vi "TempForLoop.vi"() -> ()   [LabVIEW 2015]
uses:
  <vilib>/measure/NI_MABase.lvlib
panel:
  out "Hot Temp Change":dbl
  out "Intermediate Temp Change":dbl
  out "Cold Temp Change":dbl
  out "Temperature Changes":cluster{dbl, dbl, dbl}(graph)
  out "Temperature Plot":T1(graph)
  out "Temp Data":T2
  in  "Initial Condition":T3
  in  "?":dbl
  in  "?":dbl
  # "Input desired duration of measurements in seconds"
  # "Input desired Time Measurement Intervals in seconds"
  # "Temperature Change Every Second"
  # "sec"
  # "Deg F"
  # "Deg F"
  # "Deg F"
  # "sed"
  # "Deg F"
  # "Deg F"
  # "Deg F"
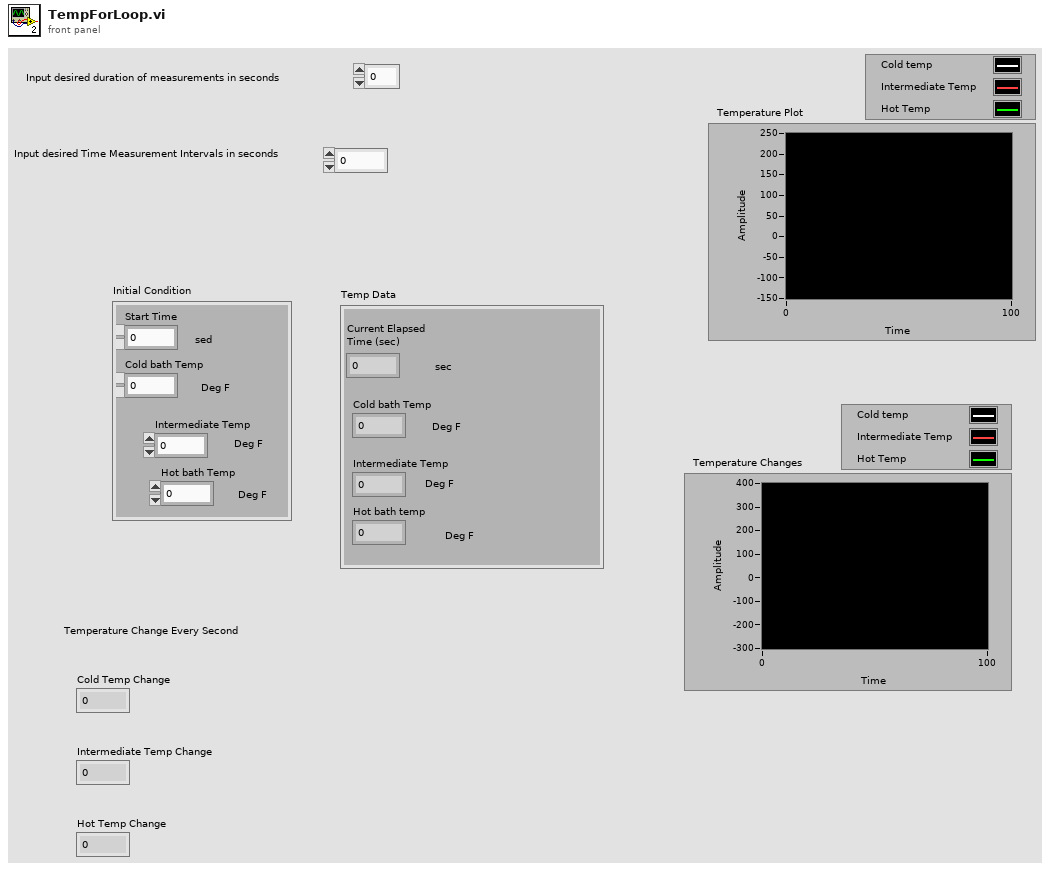
[diagram p1: front panel]
types:
  T1 = cluster{"Cold bath Temp":dbl, "Intermediate Temp":dbl, "Hot bath Temp":dbl}
  T2 = cluster{"Current Elapsed \nTime (sec)":dbl, "Cold bath Temp":dbl, "Intermediate Temp":dbl, "Hot bath temp":dbl}
  T3 = cluster{"Start Time":dbl, "Cold bath Temp":dbl, "Intermediate Temp":dbl, "Hot bath Temp":dbl}
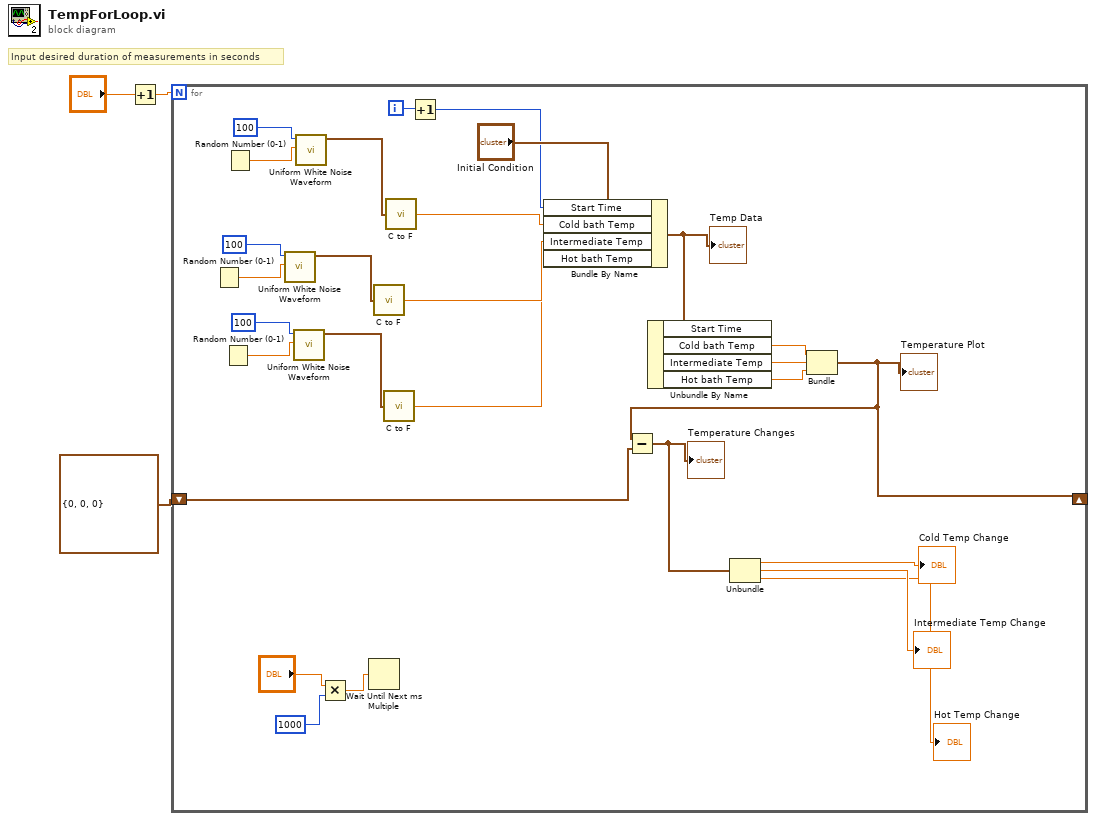
[diagram p0: block diagram]
diagram:
  # "Input desired duration of measurements in seconds"
  n1 = Increment(x="?") -> (x+1=w2:dbl)
  n2 = for {
    N: w2 -> [_]
    shift-right: [w8] -> _
    shift-left: cluster{i32, i32, i32} {0, 0, 0} -> [w9]
    i -> [w18]
    n3 = Random Number (0-1)() -> (number: 0 to 1=w26:dbl)
    n4 = Random Number (0-1)() -> (number: 0 to 1=w24:dbl)
    n5 = Random Number (0-1)() -> (number: 0 to 1=w31:dbl)
    n6 = call <vilib>:"Uniform White Noise Waveform.vi"("seed"=w26, "amplitude"=100) -> ("signal out"=w21:waveform(dbl))  [unwired: 8 in, 1 out]
    n7 = call <vilib>:"Uniform White Noise Waveform.vi"("seed"=w24, "amplitude"=100) -> ("signal out"=w20:waveform(dbl))  [unwired: 8 in, 1 out]
    n8 = call <vilib>:"Uniform White Noise Waveform.vi"("seed"=w31, "amplitude"=100) -> ("signal out"=w22:waveform(dbl))  [unwired: 8 in, 1 out]
    n9 = Multiply(x="?", y=1000) -> (x*y=w27:dbl)
    n10 = Wait Until Next ms Multiple(millisecond multiple=w27) -> ()  [unwired: 1 out]
    n11 = call "C to F.vi"("DEG C"=w21) -> ("Deg F"=w15:dbl)
    n12 = call "C to F.vi"("DEG C"=w20) -> ("Deg F"=w14:dbl)
    n13 = call "C to F.vi"("DEG C"=w22) -> ("Deg F"=w16:dbl)
    n14 = Increment(x=w18) -> (x+1=w17:i32)
    n15 = Bundle By Name(cluster="Initial Condition", "Start Time"=w17, "Cold bath Temp"=w16, "Intermediate Temp"=w15, "Hot bath Temp"=w14) -> (w13:T3)
    "Temp Data" <- w13
    n16 = Unbundle By Name(w13) -> ("Cold bath Temp"=w12:dbl, "Intermediate Temp"=w11:dbl, "Hot bath Temp"=w10:dbl)  [unwired: 1 out]
    n17 = Bundle("Cold bath Temp"=w12, "Intermediate Temp"=w11, "Hot bath Temp"=w10) -> (w8:T1)  [unwired: 1 in]
    "Temperature Plot" <- w8
    n18 = Subtract(x=w8, y=w9) -> (x-y=w7:T1)
    "Temperature Changes" <- w7
    n19 = Unbundle(w7) -> ("Cold bath Temp"=→"Cold Temp Change":dbl, "Intermediate Temp"=→"Intermediate Temp Change":dbl, "Hot bath Temp"=→"Hot Temp Change":dbl)
  }
